vi "Write Protocol.vi"(8 "error in (no error)":errorcluster, 10 "Protocol":T1, 11 "navX - SERIAL in":refnum<class "navX - SERIAL.lvclass">) -> (0 "error out":errorcluster, 3 "navX - SERIAL out":refnum<class "navX - SERIAL.lvclass">)   [LabVIEW 2015, in "navX Library v3.lvlib" / "navX - SERIAL.lvclass"]
uses:
  navX - SERIAL.lvclass
  Protocol.ctl
  navX - SERIAL.lvclass/navX - SERIAL.ctl
  navX - Interface/_TypeDefs/NotificationActionsTypeDef.ctl
  navX - Interface/navX - Interface.lvclass
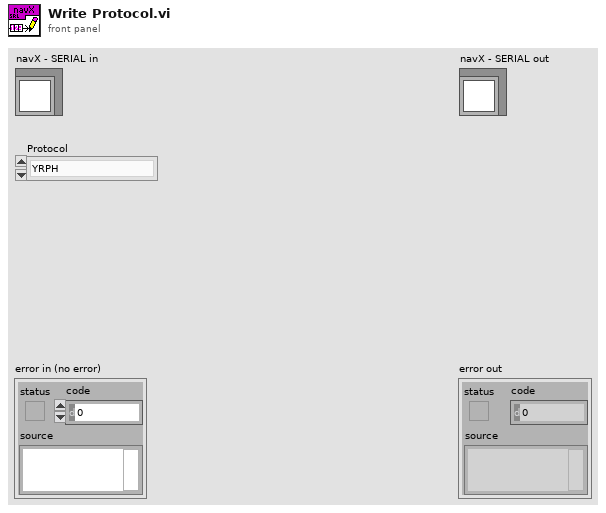
[diagram p1: front panel]
types:
  T1 = typedef "navX Library v3.lvlib/navX - SERIAL.lvclass/Protocol.ctl" = enum16{"YRPH", "Quaterinons", "Gyro/Raw", "AHRS", "AHRSAndPositioning"}
  T2 = typedef "navX Library v3.lvlib/navX - Interface.lvclass/NotificationActionsTypeDef.ctl" = enum16{"UNKNOWN", "Stop Processing Loop", "Reconfigure", "Zero"}
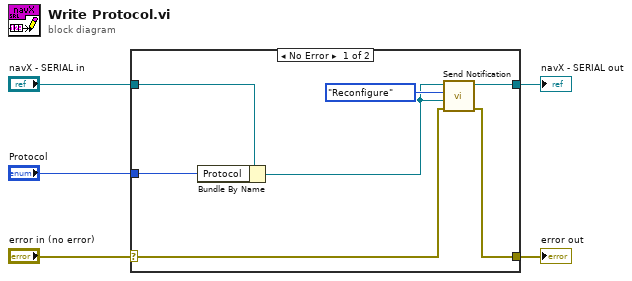
[diagram p0: block diagram]
diagram:
  n1 = case shown="No Error" "error in (no error)" {
    selector: "error in (no error)" -> [w9 w13]
    tunnel: [w8 w13] -> w4
    tunnel: [w6 w14] -> w2
    tunnel: "navX - SERIAL in" -> [w12 w14]
    tunnel: "Protocol" -> [w11 _]
    frame No Error {
      n2 = Bundle By Name(cluster=w12, "Protocol"=w11) -> (w7:refnum<class "navX - SERIAL.lvclass">)
      n3 = call "Send Notification.vi"("error in (no error)"=w9, "Notification Data"=w7, "Notification Action"=NotificationActionsTypeDef."Reconfigure", "navX - Interface in"=w7) -> ("error out"=w8:errorcluster, "navX - Interface out"=w6:refnum<class "navX - SERIAL.lvclass">)  [unwired: 6 in]
    }
    frame Error {
    }
  }
  "error out" <- w4
  "navX - SERIAL out" <- w2
